vi "AlliGator Get-Set Decay Preprocessing Parameters.vi"(6 "Get (F)/Set":bool, 8 "Error In":errorcluster, 11 "Decay Preprocessing Parameters in":T1={"Background Subtraction"=FALSE, "Straighten Decay"=FALSE, "Reverse Gates"=FALSE, "1-Normalized Decay"=FALSE, "Smoothen Decay"=FALSE, "Smoothing Parameter"=0.0, "Shift Decay"=FALSE, "Decay Shift Parameters"={"Type"=enum."Default", "Shift"=0.0, "Threshold"=0.0, "Rotate"=FALSE}, "Extrapolate Decay"=FALSE, "Additional Points"=0, "Head Fraction"=0.0, "Pixel-Normalize Decay"=FALSE, "Use Periodicity"=FALSE, "Use Cursors"=FALSE, "Tail Fraction"=0.0, "Use Decay Pre-Processing"=TRUE, "Fold Decay"=FALSE, "# Folds"=1, "[0-1]-Normalized Decay"=FALSE} {"# Folds" min=1}) -> (0 "Error Out":errorcluster, 3 "Decay Preprocessing Parameters out":T1={"Background Subtraction"=FALSE, "Straighten Decay"=FALSE, "Reverse Gates"=FALSE, "1-Normalized Decay"=FALSE, "Smoothen Decay"=FALSE, "Smoothing Parameter"=0.0, "Shift Decay"=FALSE, "Decay Shift Parameters"={"Type"=enum."Default", "Shift"=0.0, "Threshold"=0.0, "Rotate"=FALSE}, "Extrapolate Decay"=FALSE, "Additional Points"=0, "Head Fraction"=0.0, "Pixel-Normalize Decay"=FALSE, "Use Periodicity"=FALSE, "Use Cursors"=FALSE, "Tail Fraction"=0.0, "Use Decay Pre-Processing"=TRUE, "Fold Decay"=FALSE, "# Folds"=1, "[0-1]-Normalized Decay"=FALSE} {"# Folds" min=1})   [LabVIEW 2021, in "AlliGator Decay Analysis.lvlib" / "AlliGator Decay Preprocessing.lvlib"]
doc: "Get/Set Decay Pre-processing parameters."
uses:
  AlliGator Decay Preprocessing.lvlib
  AlliGator Decay Preprocessing Parameters.ctl
  Graphs/XY Graph/XY Graph Plot Shift Parameters.ctl
  Graphs/XY Graph/XY Graph Plot Shift Method.ctl
  AlliGator Settings List.ctl
  AlliGator Settings.lvlib
  Graphs/XY Graph/XY Graph Add-Ons.lvlib
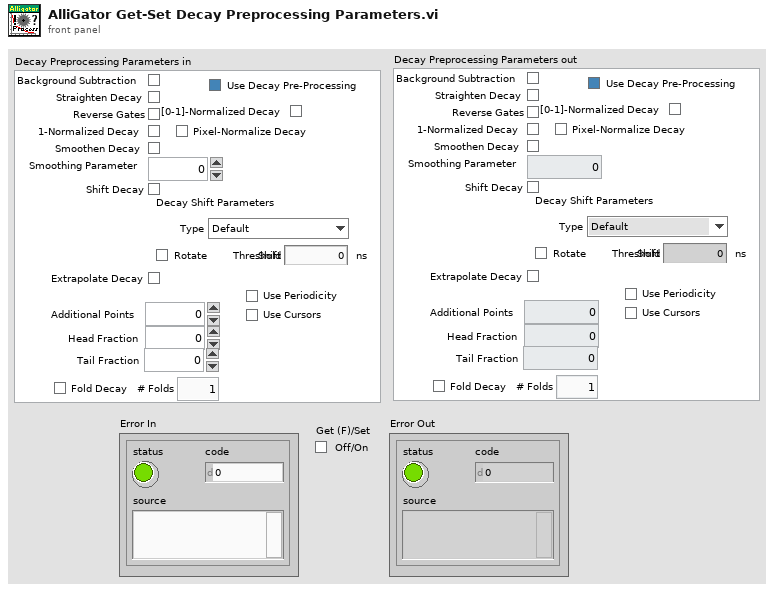
[diagram p1: front panel]
types:
  T1 = typedef "AlliGator Decay Analysis.lvlib/AlliGator Decay Preprocessing.lvlib/AlliGator Decay Preprocessing Parameters.ctl" = cluster{"Background Subtraction":bool, "Straighten Decay":bool, "Reverse Gates":bool, "1-Normalized Decay":bool, "Smoothen Decay":bool, "Smoothing Parameter":dbl, "Shift Decay":bool, "Decay Shift Parameters":T2, "Extrapolate Decay":bool, "Additional Points":u32, "Head Fraction":dbl, "Pixel-Normalize Decay":bool, "Use Periodicity":bool, "Use Cursors":bool, "Tail Fraction":dbl, "Use Decay Pre-Processing":bool, "Fold Decay":bool, "# Folds":u32, "[0-1]-Normalized Decay":bool}
  T2 = typedef "XY Graph Add-Ons.lvlib/XY Graph Plot Shift Parameters.ctl" = cluster{"Type":T3, "Shift":dbl[unit], "Threshold":dbl, "Rotate":bool}
  T3 = typedef "XY Graph Add-Ons.lvlib/XY Graph Plot Shift Method.ctl" = enum16{"Default", "CFD", "Threshold", "Cross-Correlation"}
  T4 = typedef "AlliGator Settings.lvlib/AlliGator Settings List.ctl" = enum16{"GUI:Visible Settings Tab", "GUI:Last Run Version", "Source Image:Use Image Histogram for Contrast", "Source Image:Low Count Pixels Rejection Options", "Source Image:High Count Pixels Rejection Options", "Source Image:Use Image Brightness", "Source Image:Blend Overlay with Image Background", "Source Image:Use Fixed ROI Diameter", "Source Image:ROI Diameter", "Source Image:ROI Center Color", "Source Image:Peak Threshold", "Source Image:Intensity Threshold", "Source Image:Image Binning Options", "Source Image:Image Smoothing Options", "Source Image:Image Histogram Active", "Source Image:Invert Binary Mask", "Source Image:Hot Pixel Removal", "Source Image:Overlay Analyzed ROI Center", "Source Image:Auto-Adjust Contrast", "Source Image:Histogram Lower Percentile", "Source Image:Histogram Upper Percentile", "Source Image:Save Source Image", "Source Image:Scale Bar Options", "Source Image:Image Resolution (Pixel Size)", "Data Information:Gate Width", "Data Information:Nanotime Gate Separation", "Data Information:Macrotime Gate Separation", "Data Information:Gate Step", "Data Information:# Gates", "Data Information:Gate Image Exposure", "Data Information:Gate Image Integration", "Data Information:Gates to Skip", "Data Information:Gates to Keep", "Data Information:Define Gates to", "Data Information:Channel Name", "Data Information:Available Channel Names", "Data Information:Channel Arithmetic", "Data Information:Background File Subtraction", "Data Information:Background File", "Data Information:Background Scaling Factor", "Data Information:Background Pile-up Correction", "Data Information:Background Pixel Well Capacity", "Data Information:Laser Period", "Data Information:SYNC Period", "Data Information:Pile-up Correction", "Data Information:Pixel Well Capacity", "Data Information:Dataset Scaling Factor", "Fluorescence Decay_Decay Pre-Processing:Reverse Gates", "Fluorescence Decay_Decay Pre-Processing:Verbose Decay Pre-Processing", "Fluorescence Decay_Decay Pre-Processing:Use Decay Pre-Processing", "Fluorescence Decay_Decay Pre-Processing:Background Subtraction", "Fluorescence Decay_Decay Pre-Processing:Background Definition Range", "Fluorescence Decay_Decay Pre-Processing:Baseline Subtraction Method", "Fluorescence Decay_Decay Pre-Processing:Operations Order", "Fluorescence Decay_Decay Pre-Processing:Smoothing Parameter", "Fluorescence Decay_Decay Pre-Processing:Shift Decay", "Fluorescence Decay_Decay Pre-Processing:Decay Shift Parameters", "Fluorescence Decay_Decay Pre-Processing:Fold Decay", "Fluorescence Decay_Decay Pre-Processing:# Folds", "Fluorescence Decay_Decay Pre-Processing:1-Normalize Decay", "Fluorescence Decay_Decay Pre-Processing:[0-1]-Normalize Decay", "Fluorescence Decay_Decay Pre-Processing:Smoothen Decay", "Fluorescence Decay_Decay Pre-Processing:Extrapolate Decay", "Fluorescence Decay_Decay Pre-Processing:Use Periodicity", "Fluorescence Decay_Decay Pre-Processing:Use Cursors", "Fluorescence Decay_Decay Pre-Processing:Tail Fraction", "Fluorescence Decay_Decay Pre-Processing:Head Fraction", "Fluorescence Decay_Decay Pre-Processing:Additional Points", "Fluorescence Decay_Decay Pre-Processing:Straighten Decay", "Fluorescence Decay_Decay Pre-Processing:Constant Background", "Fluorescence Decay_Decay Pre-Processing:Pixel-Normalize Decay", "Fluorescence Decay_Advanced Analysis:Extract IRF instead of Decay", "Fluorescence Decay_Advanced Analysis:IRF Extraction Options", "Fluorescence Decay_Advanced Analysis:IRF Optimization Options", "Fluorescence Decay_Advanced Analysis:Square Pulse Options", "Fluorescence Decay_Advanced Analysis:IRF Order", "Fluorescence Decay_Advanced Analysis:IRF Time Constants", "Fluorescence Decay_Advanced Analysis:Wavelet Analysis Options", "Fluorescence Decay_Advanced Analysis:Average Lifetime Options", "Fluorescence Decay_Fit Options:Fit Options", "Fluorescence Decay_Fit Options:Use Legacy Fitting Approach", "Fluorescence Decay_Fit Options:Use Data Information Laser Period", "Fluorescence Decay_Fit Parameters:Displayed Fit Parameters", "Fluorescence Decay_Fit Parameters:Fit Parameter Constraints", "Fluorescence Decay_Fit Parameters:Export Tabulated Results", "Fluorescence Decay_Fit Parameters:MLE Baseline Offset Type", "Fluorescence Decay_Fit Parameters:MLE Baseline Offset", "Fluorescence Decay_Fit Parameters:Guess Parameter Names", "Fluorescence Decay_Fit Parameters:Guess Parameter Values", "Fluorescence Decay_Fit Parameters:Guess Parameters Options", "Fluorescence Decay_Styles:Show Last Decay Only", "Fluorescence Decay_Styles:Decay Graph Color Array", "Fluorescence Decay:Decay Graph Active", "Fluorescence Decay Statistics:Min Peak Value", "Fluorescence Decay Statistics:Reject Low Decay Peak Pixels", "Fluorescence Decay Statistics:Reject High Decay Peak Pixels", "Fluorescence Decay Statistics:Max Peak Value", "Time Traces:Use File Timestamp", "Time Traces:Time Step", "Time Traces:Use Intensity Correction File", "Time Traces:Intensity Correction File", "Phasor Plot:Phasor Plot Smoothing Options", "Phasor Plot:Phasor Plot Size", "Phasor Plot:Phasor Plot Graphics Options", "Phasor Plot:Cumulative Phasor Plot", "Phasor Plot:Use Phasor Brightness", "Phasor Plot:Blend Overlay with Phasor Background", "Phasor Plot:Save Phasor Plot", "Phasor Plot:Show References", "Phasor Plot:Phasor Ratio Decay Range", "Phasor Plot:Exponential Fading", "Phasor Plot:Phasor Ratio Reference Colors", "Phasor Plot:Reference Radius", "Phasor Plot:Show Color Map Vertices", "Phasor Plot:Phasor Plot Active", "Phasor Plot:Phasor Ratio Color Map Type", "Phasor Plot:Phasor Ratio Color Map", "Phasor Plot:Phasor Ratio Display Range", "Phasor Plot:Selected Image ROI(s)", "Phasor Plot:All Image ROIs", "Phasor Plot:Selected Phasor Plot ROI(s)", "Phasor Plot:All Phasor Plot ROIs", "Phasor Plot:Phasor Ratio Color-Coded Quantity", "Phasor Plot:Store Phasor Harmonics", "Phasor Plot:Draw Reference Segment", "Phasor Plot:User-Defined Quantity", "Phasor Graph:Phasor Frequency", "Phasor Graph:Phasor Ratio Type", "Phasor Graph:Pixel-level Phasor Computation", "Phasor Graph:Save Phasor Graph", "Phasor Graph:Phasor Graph Active", "Phasor Graph:Phasor SDV Options", "Phasor Calibration:Use Backup Calibration if needed", "Phasor Graph:Define Shortest Lifetime as", "Phasor Calibration:Backup Calibration Type", "Phasor Calibration:Calibration Type", "Phasor Calibration:Calibration Lifetime", "Phasor Calibration:Calibration Map Algorithm", "Single-Exponential Phasor Locus (SEPL):Gate Parameters", "Single-Exponential Phasor Locus (SEPL):User-defined Gate", "Single-Exponential Phasor Locus (SEPL):User-defined IRF", "Single-Exponential Phasor Locus (SEPL):Phasor Parameters", "Single-Exponential Phasor Locus (SEPL):Decay & IRF Parameters", "Single-Exponential Phasor Locus (SEPL):Display Parameters", "Lifetime Analysis:Decay Analysis Parameters", "Lifetime Analysis:Lifetime Map Active", "Plugins:Python Settings", "Miscellaneous:Verbose Mode", "Miscellaneous:Beep after Script", "Miscellaneous:Saved Image File Format", "Miscellaneous:Exported Gate Image Settings", "Miscellaneous:Include Loading in Timing", "Miscellaneous:Verbose Settings Mode", "Miscellaneous:Histogram Options", "Miscellaneous:Beep on Error", "Miscellaneous:# Logical Processors Used", "Miscellaneous:ROI Description Max Characters", "Miscellaneous:Verbose Error Mode", "Miscellaneous:Transparent Mask Color"}
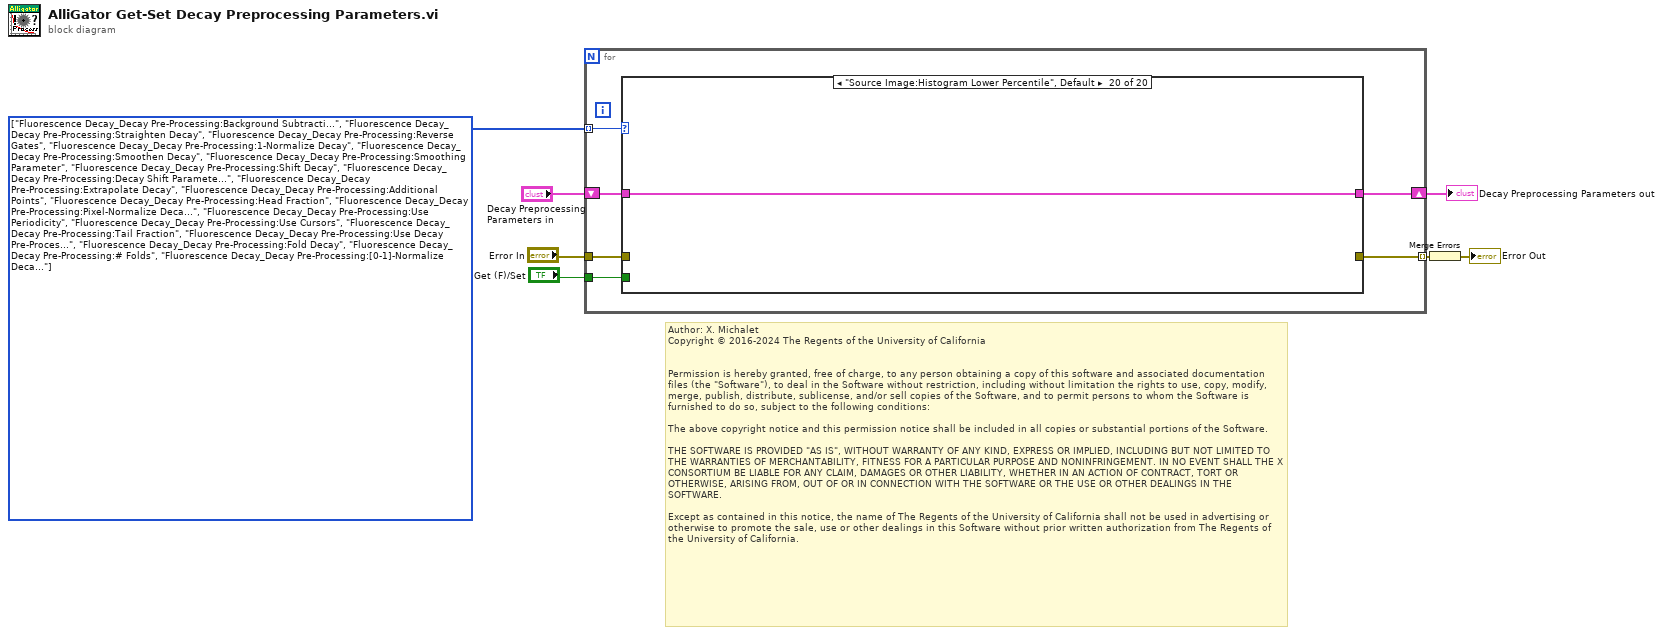
[diagram p0: block diagram]
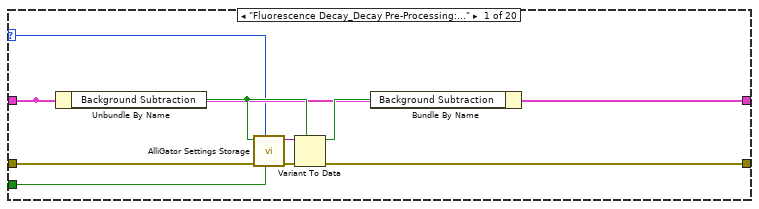
[diagram p2: hidden frame]
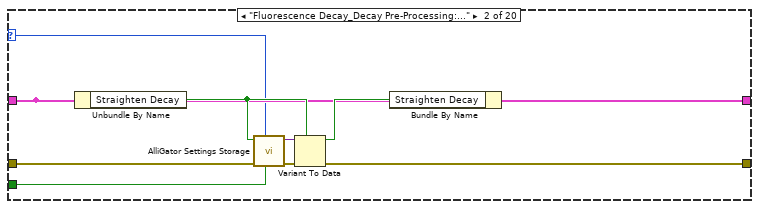
[diagram p3: hidden frame]
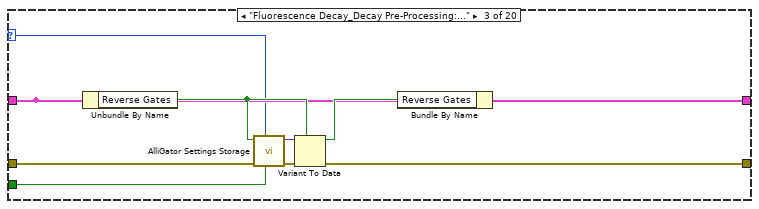
[diagram p4: hidden frame]
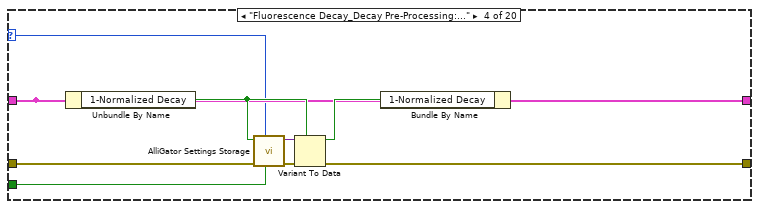
[diagram p5: hidden frame]
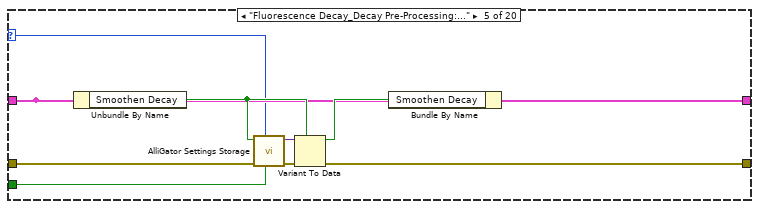
[diagram p6: hidden frame]
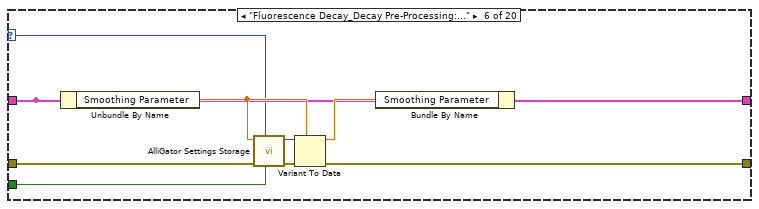
[diagram p7: hidden frame]
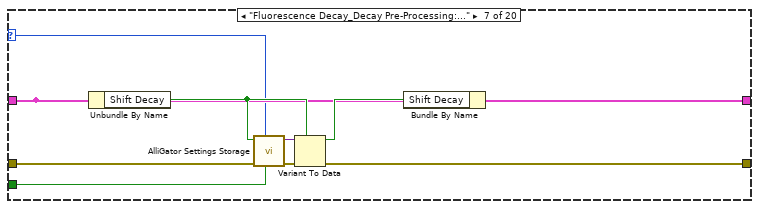
[diagram p8: hidden frame]
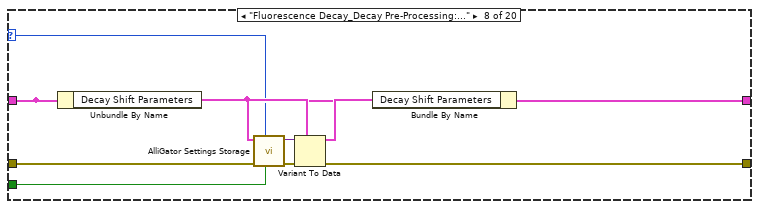
[diagram p9: hidden frame]
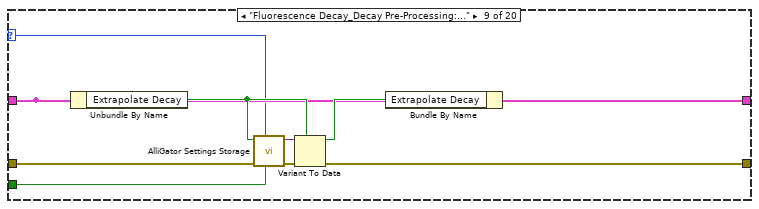
[diagram p10: hidden frame]
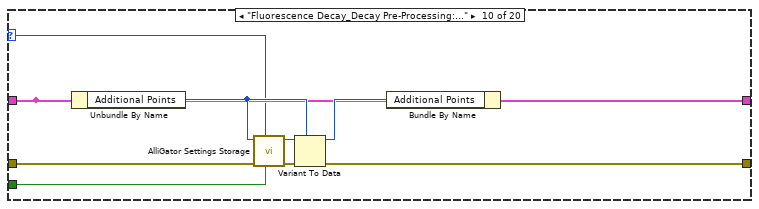
[diagram p11: hidden frame]
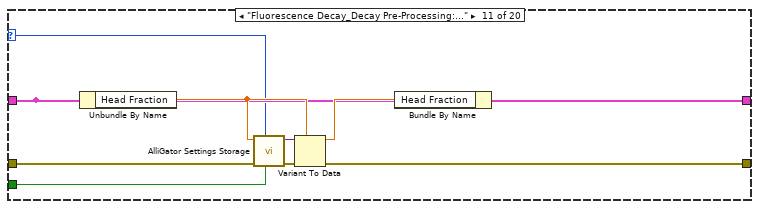
[diagram p12: hidden frame]
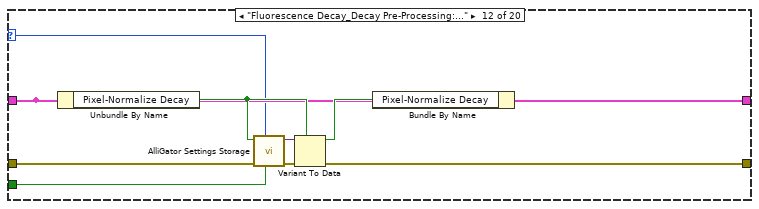
[diagram p13: hidden frame]
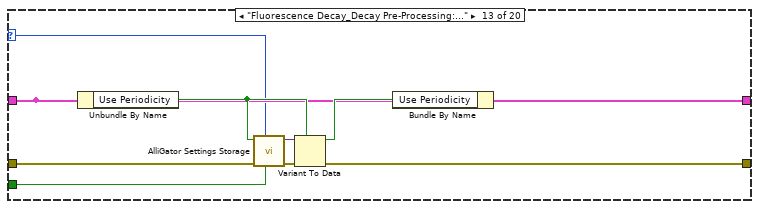
[diagram p14: hidden frame]
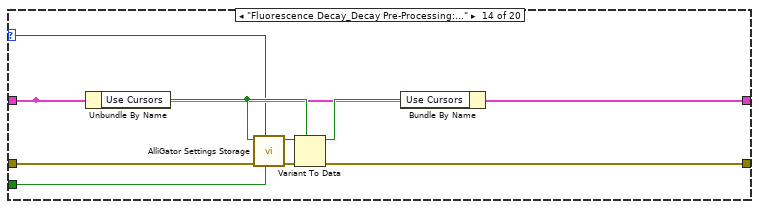
[diagram p15: hidden frame]
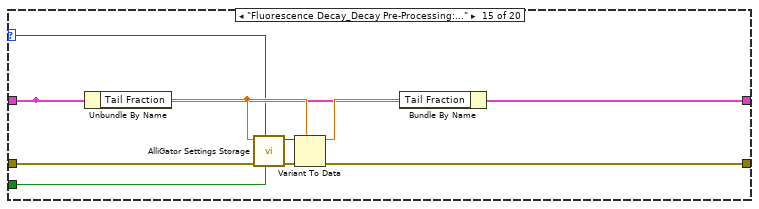
[diagram p16: hidden frame]
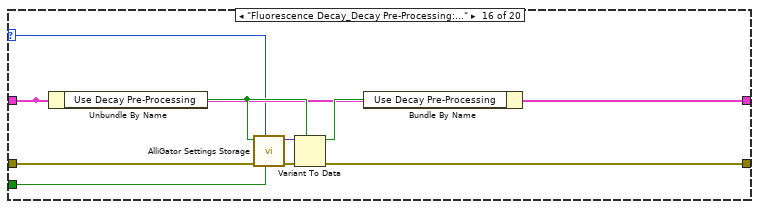
[diagram p17: hidden frame]
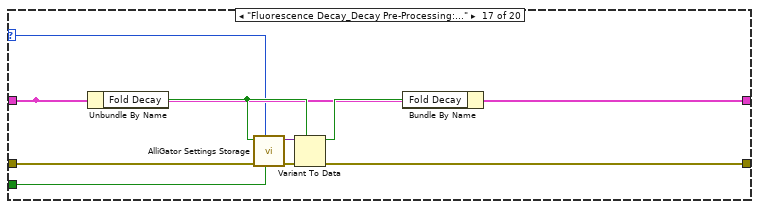
[diagram p18: hidden frame]
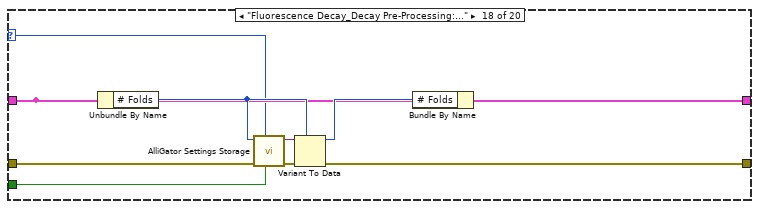
[diagram p19: hidden frame]
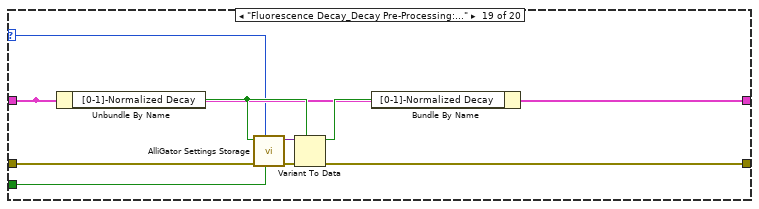
[diagram p20: hidden frame]
diagram:
  w1 = T4[] [enum."Fluorescence Decay_Decay Pre-Processing:Background Subtraction", enum."Fluorescence Decay_Decay Pre-Processing:Straighten Decay", enum."Fluorescence Decay_Decay Pre-Processing:Reverse Gates", enum."Fluorescence Decay_Decay Pre-Processing:1-Normalize Decay", enum."Fluorescence Decay_Decay Pre-Processing:Smoothen Decay", enum."Fluorescence Decay_Decay Pre-Processing:Smoothing Parameter", enum."Fluorescence Decay_Decay Pre-Processing:Shift Decay", enum."Fluorescence Decay_Decay Pre-Processing:Decay Shift Parameters", enum."Fluorescence Decay_Decay Pre-Processing:Extrapolate Decay", enum."Fluorescence Decay_Decay Pre-Processing:Additional Points", enum."Fluorescence Decay_Decay Pre-Processing:Head Fraction", enum."Fluorescence Decay_Decay Pre-Processing:Pixel-Normalize Decay", enum."Fluorescence Decay_Decay Pre-Processing:Use Periodicity", enum."Fluorescence Decay_Decay Pre-Processing:Use Cursors", enum."Fluorescence Decay_Decay Pre-Processing:Tail Fraction", enum."Fluorescence Decay_Decay Pre-Processing:Use Decay Pre-Processing", enum."Fluorescence Decay_Decay Pre-Processing:Fold Decay", enum."Fluorescence Decay_Decay Pre-Processing:# Folds", enum."Fluorescence Decay_Decay Pre-Processing:[0-1]-Normalize Decay"] items=["GUI:Visible Settings Tab", "GUI:Last Run Version", "Source Image:Use Image Histogram for Contrast", "Source Image:Low Count Pixels Rejection Options", "Source Image:High Count Pixels Rejection Options", "Source Image:Use Image Brightness", "Source Image:Blend Overlay with Image Background", "Source Image:Use Fixed ROI Diameter", "Source Image:ROI Diameter", "Source Image:ROI Center Color", "Source Image:Peak Threshold", "Source Image:Intensity Threshold", "Source Image:Image Binning Options", "Source Image:Image Smoothing Options", "Source Image:Image Histogram Active", "Source Image:Invert Binary Mask", "Source Image:Hot Pixel Removal", "Source Image:Overlay Analyzed ROI Center", "Source Image:Auto-Adjust Contrast", "Source Image:Histogram Lower Percentile", "Source Image:Histogram Upper Percentile", "Source Image:Save Source Image", "Source Image:Scale Bar Options", "Source Image:Image Resolution (Pixel Size)", "Data Information:Gate Width", "Data Information:Nanotime Gate Separation", "Data Information:Macrotime Gate Separation", "Data Information:Gate Step", "Data Information:# Gates", "Data Information:Gate Image Exposure", "Data Information:Gate Image Integration", "Data Information:Gates to Skip", "Data Information:Gates to Keep", "Data Information:Define Gates to", "Data Information:Channel Name", "Data Information:Available Channel Names", "Data Information:Channel Arithmetic", "Data Information:Background File Subtraction", "Data Information:Background File", "Data Information:Background Scaling Factor", "Data Information:Background Pile-up Correction", "Data Information:Background Pixel Well Capacity", "Data Information:Laser Period", "Data Information:SYNC Period", "Data Information:Pile-up Correction", "Data Information:Pixel Well Capacity", "Data Information:Dataset Scaling Factor", "Fluorescence Decay_Decay Pre-Processing:Reverse Gates", "Fluorescence Decay_Decay Pre-Processing:Verbose Decay Pre-Processing", "Fluorescence Decay_Decay Pre-Processing:Use Decay Pre-Processing", "Fluorescence Decay_Decay Pre-Processing:Background Subtraction", "Fluorescence Decay_Decay Pre-Processing:Background Definition Range", "Fluorescence Decay_Decay Pre-Processing:Baseline Subtraction Method", "Fluorescence Decay_Decay Pre-Processing:Operations Order", "Fluorescence Decay_Decay Pre-Processing:Smoothing Parameter", "Fluorescence Decay_Decay Pre-Processing:Shift Decay", "Fluorescence Decay_Decay Pre-Processing:Decay Shift Parameters", "Fluorescence Decay_Decay Pre-Processing:Fold Decay", "Fluorescence Decay_Decay Pre-Processing:# Folds", "Fluorescence Decay_Decay Pre-Processing:1-Normalize Decay", "Fluorescence Decay_Decay Pre-Processing:[0-1]-Normalize Decay", "Fluorescence Decay_Decay Pre-Processing:Smoothen Decay", "Fluorescence Decay_Decay Pre-Processing:Extrapolate Decay", "Fluorescence Decay_Decay Pre-Processing:Use Periodicity", "Fluorescence Decay_Decay Pre-Processing:Use Cursors", "Fluorescence Decay_Decay Pre-Processing:Tail Fraction", "Fluorescence Decay_Decay Pre-Processing:Head Fraction", "Fluorescence Decay_Decay Pre-Processing:Additional Points", "Fluorescence Decay_Decay Pre-Processing:Straighten Decay", "Fluorescence Decay_Decay Pre-Processing:Constant Background", "Fluorescence Decay_Decay Pre-Processing:Pixel-Normalize Decay", "Fluorescence Decay_Advanced Analysis:Extract IRF instead of Decay", "Fluorescence Decay_Advanced Analysis:IRF Extraction Options", "Fluorescence Decay_Advanced Analysis:IRF Optimization Options", "Fluorescence Decay_Advanced Analysis:Square Pulse Options", "Fluorescence Decay_Advanced Analysis:IRF Order", "Fluorescence Decay_Advanced Analysis:IRF Time Constants", "Fluorescence Decay_Advanced Analysis:Wavelet Analysis Options", "Fluorescence Decay_Advanced Analysis:Average Lifetime Options", "Fluorescence Decay_Fit Options:Fit Options", "Fluorescence Decay_Fit Options:Use Legacy Fitting Approach", "Fluorescence Decay_Fit Options:Use Data Information Laser Period", "Fluorescence Decay_Fit Parameters:Displayed Fit Parameters", "Fluorescence Decay_Fit Parameters:Fit Parameter Constraints", "Fluorescence Decay_Fit Parameters:Export Tabulated Results", "Fluorescence Decay_Fit Parameters:MLE Baseline Offset Type", "Fluorescence Decay_Fit Parameters:MLE Baseline Offset", "Fluorescence Decay_Fit Parameters:Guess Parameter Names", "Fluorescence Decay_Fit Parameters:Guess Parameter Values", "Fluorescence Decay_Fit Parameters:Guess Parameters Options", "Fluorescence Decay_Styles:Show Last Decay Only", "Fluorescence Decay_Styles:Decay Graph Color Array", "Fluorescence Decay:Decay Graph Active", "Fluorescence Decay Statistics:Min Peak Value", "Fluorescence Decay Statistics:Reject Low Decay Peak Pixels", "Fluorescence Decay Statistics:Reject High Decay Peak Pixels", "Fluorescence Decay Statistics:Max Peak Value", "Time Traces:Use File Timestamp", "Time Traces:Time Step", "Time Traces:Use Intensity Correction File", "Time Traces:Intensity Correction File", "Phasor Plot:Phasor Plot Smoothing Options", "Phasor Plot:Phasor Plot Size", "Phasor Plot:Phasor Plot Graphics Options", "Phasor Plot:Cumulative Phasor Plot", "Phasor Plot:Use Phasor Brightness", "Phasor Plot:Blend Overlay with Phasor Background", "Phasor Plot:Save Phasor Plot", "Phasor Plot:Show References", "Phasor Plot:Phasor Ratio Decay Range", "Phasor Plot:Exponential Fading", "Phasor Plot:Phasor Ratio Reference Colors", "Phasor Plot:Reference Radius", "Phasor Plot:Show Color Map Vertices", "Phasor Plot:Phasor Plot Active", "Phasor Plot:Phasor Ratio Color Map Type", "Phasor Plot:Phasor Ratio Color Map", "Phasor Plot:Phasor Ratio Display Range", "Phasor Plot:Selected Image ROI(s)", "Phasor Plot:All Image ROIs", "Phasor Plot:Selected Phasor Plot ROI(s)", "Phasor Plot:All Phasor Plot ROIs", "Phasor Plot:Phasor Ratio Color-Coded Quantity", "Phasor Plot:Store Phasor Harmonics", "Phasor Plot:Draw Reference Segment", "Phasor Plot:User-Defined Quantity", "Phasor Graph:Phasor Frequency", "Phasor Graph:Phasor Ratio Type", "Phasor Graph:Pixel-level Phasor Computation", "Phasor Graph:Save Phasor Graph", "Phasor Graph:Phasor Graph Active", "Phasor Graph:Phasor SDV Options", "Phasor Calibration:Use Backup Calibration if needed", "Phasor Graph:Define Shortest Lifetime as", "Phasor Calibration:Backup Calibration Type", "Phasor Calibration:Calibration Type", "Phasor Calibration:Calibration Lifetime", "Phasor Calibration:Calibration Map Algorithm", "Single-Exponential Phasor Locus (SEPL):Gate Parameters", "Single-Exponential Phasor Locus (SEPL):User-defined Gate", "Single-Exponential Phasor Locus (SEPL):User-defined IRF", "Single-Exponential Phasor Locus (SEPL):Phasor Parameters", "Single-Exponential Phasor Locus (SEPL):Decay & IRF Parameters", "Single-Exponential Phasor Locus (SEPL):Display Parameters", "Lifetime Analysis:Decay Analysis Parameters", "Lifetime Analysis:Lifetime Map Active", "Plugins:Python Settings", "Miscellaneous:Verbose Mode", "Miscellaneous:Beep after Script", "Miscellaneous:Saved Image File Format", "Miscellaneous:Exported Gate Image Settings", "Miscellaneous:Include Loading in Timing", "Miscellaneous:Verbose Settings Mode", "Miscellaneous:Histogram Options", "Miscellaneous:Beep on Error", "Miscellaneous:# Logical Processors Used", "Miscellaneous:ROI Description Max Characters", "Miscellaneous:Verbose Error Mode", "Miscellaneous:Transparent Mask Color"] ("Array")
  # "Author: X. Michalet\nCopyright © 2016-2024 The Regents of the University of California\n \n\nPermission is hereby granted, free of charge, to any person obtaining a copy of this software and associated documentation files (the \"Software\"), to deal in the Software without restriction, including without limitation the rights to use, copy, modify, merge, publish, distribute, sublicense, and/or sell copies of the Software, and to permit persons to whom the Software is furnished to do so, subject to the following conditions:\n\nThe above copyright notice and this permission notice shall be included in all copies or substantial portions of the Software.\n\nTHE SOFTWARE IS PROVIDED \"AS IS\", WITHOUT WARRANTY OF ANY KIND, EXPRESS OR IMPLIED, INCLUDING BUT NOT LIMITED TO THE WARRANTIES OF MERCHANTABILITY, FITNESS FOR A PARTICULAR PURPOSE AND NONINFRINGEMENT. IN NO EVENT SHALL THE X CONSORTIUM BE LIABLE FOR ANY CLAIM, DAMAGES OR OTHER LIABILITY, WHETHER IN AN ACTION OF CONTRACT, TORT OR OTHERWISE, ARISING FROM, OUT OF OR IN CONNECTION WITH THE SOFTWARE OR THE USE OR OTHER DEALINGS IN THE SOFTWARE.\n\nExcept as contained in this notice, the name of The Regents of the University of California shall not be used in advertising or otherwise to promote the sale, use or other dealings in this Software without prior written authorization from The Regents of the University of California."
  n1 = for {
    tunnel: "Get (F)/Set" -> [w11]
    shift-right: [w12] -> w7
    shift-left: "Decay Preprocessing Parameters in" -> [w13]
    tunnel: "Error In" -> [w10]
    tunnel: [w9] -> w3 mode=indexing
    tunnel: w1 -> [w8] mode=indexing
    n2 = case shown="\"Source Image:Histogram Lower Percentile\", Default" w8 {
      selector: w8 -> [w14 w24 w34 w44 w54 w64 w74 w84 w94 w104 w114 w124 w134 w144 w154 w164 w174 w184 w194 _]
      tunnel: w13 -> [w15 w25 w35 w45 w55 w65 w75 w85 w95 w105 w115 w125 w135 w145 w155 w165 w175 w185 w195 w204]
      tunnel: [w19 w29 w39 w49 w59 w69 w79 w89 w99 w109 w119 w129 w139 w149 w159 w169 w179 w189 w199 w204] -> w12
      tunnel: w11 -> [w18 w28 w38 w48 w58 w68 w78 w88 w98 w108 w118 w128 w138 w148 w158 w168 w178 w188 w198 _]
      tunnel: w10 -> [w17 w27 w37 w47 w57 w67 w77 w87 w97 w107 w117 w127 w137 w147 w157 w167 w177 w187 w197 _]
      tunnel: [w16 w26 w36 w46 w56 w66 w76 w86 w96 w106 w116 w126 w136 w146 w156 w166 w176 w186 w196 _] -> w9
      frame "Fluorescence Decay_Decay Pre-Processing:Background Subtraction" {
        n3 = Unbundle By Name(w15) -> ("Background Subtraction"=w20:bool)
        n4 = call "AlliGator Settings Storage.vi"("Get(F)/Set"=w18, "AlliGator Settings List"=w14, "Error In"=w17, "Variant Data in"=w20) -> ("Error Out"=w23:errorcluster, "Variant Data out"=w22:variant)  [unwired: 6 in]
        n5 = Variant To Data(error in=w23, type=w20, Variant=w22) -> (data=w21:bool, error out=w16:errorcluster)
        n6 = Bundle By Name(cluster=w15, "Background Subtraction"=w21) -> (w19:T1)
      }
      frame "Fluorescence Decay_Decay Pre-Processing:Straighten Decay" {
        n7 = Unbundle By Name(w25) -> ("Straighten Decay"=w30:bool)
        n8 = call "AlliGator Settings Storage.vi"("Get(F)/Set"=w28, "AlliGator Settings List"=w24, "Error In"=w27, "Variant Data in"=w30) -> ("Error Out"=w33:errorcluster, "Variant Data out"=w32:variant)  [unwired: 6 in]
        n9 = Variant To Data(error in=w33, type=w30, Variant=w32) -> (data=w31:bool, error out=w26:errorcluster)
        n10 = Bundle By Name(cluster=w25, "Straighten Decay"=w31) -> (w29:T1)
      }
      frame "Fluorescence Decay_Decay Pre-Processing:Reverse Gates" {
        n11 = Unbundle By Name(w35) -> ("Reverse Gates"=w40:bool)
        n12 = call "AlliGator Settings Storage.vi"("Get(F)/Set"=w38, "AlliGator Settings List"=w34, "Error In"=w37, "Variant Data in"=w40) -> ("Error Out"=w43:errorcluster, "Variant Data out"=w42:variant)  [unwired: 6 in]
        n13 = Variant To Data(error in=w43, type=w40, Variant=w42) -> (data=w41:bool, error out=w36:errorcluster)
        n14 = Bundle By Name(cluster=w35, "Reverse Gates"=w41) -> (w39:T1)
      }
      frame "Fluorescence Decay_Decay Pre-Processing:1-Normalize Decay" {
        n15 = Unbundle By Name(w45) -> ("1-Normalized Decay"=w50:bool)
        n16 = call "AlliGator Settings Storage.vi"("Get(F)/Set"=w48, "AlliGator Settings List"=w44, "Error In"=w47, "Variant Data in"=w50) -> ("Error Out"=w53:errorcluster, "Variant Data out"=w52:variant)  [unwired: 6 in]
        n17 = Variant To Data(error in=w53, type=w50, Variant=w52) -> (data=w51:bool, error out=w46:errorcluster)
        n18 = Bundle By Name(cluster=w45, "1-Normalized Decay"=w51) -> (w49:T1)
      }
      frame "Fluorescence Decay_Decay Pre-Processing:Smoothen Decay" {
        n19 = Unbundle By Name(w55) -> ("Smoothen Decay"=w60:bool)
        n20 = call "AlliGator Settings Storage.vi"("Get(F)/Set"=w58, "AlliGator Settings List"=w54, "Error In"=w57, "Variant Data in"=w60) -> ("Error Out"=w63:errorcluster, "Variant Data out"=w62:variant)  [unwired: 6 in]
        n21 = Variant To Data(error in=w63, type=w60, Variant=w62) -> (data=w61:bool, error out=w56:errorcluster)
        n22 = Bundle By Name(cluster=w55, "Smoothen Decay"=w61) -> (w59:T1)
      }
      frame "Fluorescence Decay_Decay Pre-Processing:Smoothing Parameter" {
        n23 = Unbundle By Name(w65) -> ("Smoothing Parameter"=w70:dbl)
        n24 = call "AlliGator Settings Storage.vi"("Get(F)/Set"=w68, "AlliGator Settings List"=w64, "Error In"=w67, "Variant Data in"=w70) -> ("Error Out"=w73:errorcluster, "Variant Data out"=w72:variant)  [unwired: 6 in]
        n25 = Variant To Data(error in=w73, type=w70, Variant=w72) -> (data=w71:dbl, error out=w66:errorcluster)
        n26 = Bundle By Name(cluster=w65, "Smoothing Parameter"=w71) -> (w69:T1)
      }
      frame "Fluorescence Decay_Decay Pre-Processing:Shift Decay" {
        n27 = Unbundle By Name(w75) -> ("Shift Decay"=w80:bool)
        n28 = call "AlliGator Settings Storage.vi"("Get(F)/Set"=w78, "AlliGator Settings List"=w74, "Error In"=w77, "Variant Data in"=w80) -> ("Error Out"=w83:errorcluster, "Variant Data out"=w82:variant)  [unwired: 6 in]
        n29 = Variant To Data(error in=w83, type=w80, Variant=w82) -> (data=w81:bool, error out=w76:errorcluster)
        n30 = Bundle By Name(cluster=w75, "Shift Decay"=w81) -> (w79:T1)
      }
      frame "Fluorescence Decay_Decay Pre-Processing:Decay Shift Parameters" {
        n31 = Unbundle By Name(w85) -> ("Decay Shift Parameters"=w90:T2)
        n32 = call "AlliGator Settings Storage.vi"("Get(F)/Set"=w88, "AlliGator Settings List"=w84, "Error In"=w87, "Variant Data in"=w90) -> ("Error Out"=w93:errorcluster, "Variant Data out"=w92:variant)  [unwired: 6 in]
        n33 = Variant To Data(error in=w93, type=w90, Variant=w92) -> (data=w91:T2, error out=w86:errorcluster)
        n34 = Bundle By Name(cluster=w85, "Decay Shift Parameters"=w91) -> (w89:T1)
      }
      frame "Fluorescence Decay_Decay Pre-Processing:Extrapolate Decay" {
        n35 = Unbundle By Name(w95) -> ("Extrapolate Decay"=w100:bool)
        n36 = call "AlliGator Settings Storage.vi"("Get(F)/Set"=w98, "AlliGator Settings List"=w94, "Error In"=w97, "Variant Data in"=w100) -> ("Error Out"=w103:errorcluster, "Variant Data out"=w102:variant)  [unwired: 6 in]
        n37 = Variant To Data(error in=w103, type=w100, Variant=w102) -> (data=w101:bool, error out=w96:errorcluster)
        n38 = Bundle By Name(cluster=w95, "Extrapolate Decay"=w101) -> (w99:T1)
      }
      frame "Fluorescence Decay_Decay Pre-Processing:Additional Points" {
        n39 = Unbundle By Name(w105) -> ("Additional Points"=w110:u32)
        n40 = call "AlliGator Settings Storage.vi"("Get(F)/Set"=w108, "AlliGator Settings List"=w104, "Error In"=w107, "Variant Data in"=w110) -> ("Error Out"=w113:errorcluster, "Variant Data out"=w112:variant)  [unwired: 6 in]
        n41 = Variant To Data(error in=w113, type=w110, Variant=w112) -> (data=w111:u32, error out=w106:errorcluster)
        n42 = Bundle By Name(cluster=w105, "Additional Points"=w111) -> (w109:T1)
      }
      frame "Fluorescence Decay_Decay Pre-Processing:Head Fraction" {
        n43 = Unbundle By Name(w115) -> ("Head Fraction"=w120:dbl)
        n44 = call "AlliGator Settings Storage.vi"("Get(F)/Set"=w118, "AlliGator Settings List"=w114, "Error In"=w117, "Variant Data in"=w120) -> ("Error Out"=w123:errorcluster, "Variant Data out"=w122:variant)  [unwired: 6 in]
        n45 = Variant To Data(error in=w123, type=w120, Variant=w122) -> (data=w121:dbl, error out=w116:errorcluster)
        n46 = Bundle By Name(cluster=w115, "Head Fraction"=w121) -> (w119:T1)
      }
      frame "Fluorescence Decay_Decay Pre-Processing:Pixel-Normalize Decay" {
        n47 = Unbundle By Name(w125) -> ("Pixel-Normalize Decay"=w130:bool)
        n48 = call "AlliGator Settings Storage.vi"("Get(F)/Set"=w128, "AlliGator Settings List"=w124, "Error In"=w127, "Variant Data in"=w130) -> ("Error Out"=w133:errorcluster, "Variant Data out"=w132:variant)  [unwired: 6 in]
        n49 = Variant To Data(error in=w133, type=w130, Variant=w132) -> (data=w131:bool, error out=w126:errorcluster)
        n50 = Bundle By Name(cluster=w125, "Pixel-Normalize Decay"=w131) -> (w129:T1)
      }
      frame "Fluorescence Decay_Decay Pre-Processing:Use Periodicity" {
        n51 = Unbundle By Name(w135) -> ("Use Periodicity"=w140:bool)
        n52 = call "AlliGator Settings Storage.vi"("Get(F)/Set"=w138, "AlliGator Settings List"=w134, "Error In"=w137, "Variant Data in"=w140) -> ("Error Out"=w143:errorcluster, "Variant Data out"=w142:variant)  [unwired: 6 in]
        n53 = Variant To Data(error in=w143, type=w140, Variant=w142) -> (data=w141:bool, error out=w136:errorcluster)
        n54 = Bundle By Name(cluster=w135, "Use Periodicity"=w141) -> (w139:T1)
      }
      frame "Fluorescence Decay_Decay Pre-Processing:Use Cursors" {
        n55 = Unbundle By Name(w145) -> ("Use Cursors"=w150:bool)
        n56 = call "AlliGator Settings Storage.vi"("Get(F)/Set"=w148, "AlliGator Settings List"=w144, "Error In"=w147, "Variant Data in"=w150) -> ("Error Out"=w153:errorcluster, "Variant Data out"=w152:variant)  [unwired: 6 in]
        n57 = Variant To Data(error in=w153, type=w150, Variant=w152) -> (data=w151:bool, error out=w146:errorcluster)
        n58 = Bundle By Name(cluster=w145, "Use Cursors"=w151) -> (w149:T1)
      }
      frame "Fluorescence Decay_Decay Pre-Processing:Tail Fraction" {
        n59 = Unbundle By Name(w155) -> ("Tail Fraction"=w160:dbl)
        n60 = call "AlliGator Settings Storage.vi"("Get(F)/Set"=w158, "AlliGator Settings List"=w154, "Error In"=w157, "Variant Data in"=w160) -> ("Error Out"=w163:errorcluster, "Variant Data out"=w162:variant)  [unwired: 6 in]
        n61 = Variant To Data(error in=w163, type=w160, Variant=w162) -> (data=w161:dbl, error out=w156:errorcluster)
        n62 = Bundle By Name(cluster=w155, "Tail Fraction"=w161) -> (w159:T1)
      }
      frame "Fluorescence Decay_Decay Pre-Processing:Use Decay Pre-Processing" {
        n63 = Unbundle By Name(w165) -> ("Use Decay Pre-Processing"=w170:bool)
        n64 = call "AlliGator Settings Storage.vi"("Get(F)/Set"=w168, "AlliGator Settings List"=w164, "Error In"=w167, "Variant Data in"=w170) -> ("Error Out"=w173:errorcluster, "Variant Data out"=w172:variant)  [unwired: 6 in]
        n65 = Variant To Data(error in=w173, type=w170, Variant=w172) -> (data=w171:bool, error out=w166:errorcluster)
        n66 = Bundle By Name(cluster=w165, "Use Decay Pre-Processing"=w171) -> (w169:T1)
      }
      frame "Fluorescence Decay_Decay Pre-Processing:Fold Decay" {
        n67 = Unbundle By Name(w175) -> ("Fold Decay"=w180:bool)
        n68 = call "AlliGator Settings Storage.vi"("Get(F)/Set"=w178, "AlliGator Settings List"=w174, "Error In"=w177, "Variant Data in"=w180) -> ("Error Out"=w183:errorcluster, "Variant Data out"=w182:variant)  [unwired: 6 in]
        n69 = Variant To Data(error in=w183, type=w180, Variant=w182) -> (data=w181:bool, error out=w176:errorcluster)
        n70 = Bundle By Name(cluster=w175, "Fold Decay"=w181) -> (w179:T1)
      }
      frame "Fluorescence Decay_Decay Pre-Processing:# Folds" {
        n71 = Unbundle By Name(w185) -> ("# Folds"=w190:u32)
        n72 = call "AlliGator Settings Storage.vi"("Get(F)/Set"=w188, "AlliGator Settings List"=w184, "Error In"=w187, "Variant Data in"=w190) -> ("Error Out"=w193:errorcluster, "Variant Data out"=w192:variant)  [unwired: 6 in]
        n73 = Variant To Data(error in=w193, type=w190, Variant=w192) -> (data=w191:u32, error out=w186:errorcluster)
        n74 = Bundle By Name(cluster=w185, "# Folds"=w191) -> (w189:T1)
      }
      frame "Fluorescence Decay_Decay Pre-Processing:[0-1]-Normalize Decay" {
        n75 = Unbundle By Name(w195) -> ("[0-1]-Normalized Decay"=w200:bool)
        n76 = call "AlliGator Settings Storage.vi"("Get(F)/Set"=w198, "AlliGator Settings List"=w194, "Error In"=w197, "Variant Data in"=w200) -> ("Error Out"=w203:errorcluster, "Variant Data out"=w202:variant)  [unwired: 6 in]
        n77 = Variant To Data(error in=w203, type=w200, Variant=w202) -> (data=w201:bool, error out=w196:errorcluster)
        n78 = Bundle By Name(cluster=w195, "[0-1]-Normalized Decay"=w201) -> (w199:T1)
      }
      frame "Source Image:Histogram Lower Percentile", Default {
      }
    }
  }
  "Decay Preprocessing Parameters out" <- w7
  n79 = Merge Errors(w3) -> (→"Error Out":errorcluster)
